vi "Setup Set Cluster Values from Pathed JSON String.vi"() -> (0 "error out":errorcluster, 2 "JSON string":string="{\n\t\"Width\":640,\n\t\"Height\":480,\n\t\"Sensor\":\"A700\",\n    \"TriggerMode\":0,\n    \"TriggerSource\":1,\n    \"TriggerActivation\":0,\n    \"TriggerSelector\":0,\n    \"AcquisitionMode\":2,\n    \"OutputImageType\":7,\n    \"AcquisitionFrameRate\":1.0,\n    \"AcquisitionFrameCount\":100,\n    \"Timeout\":20000,\n    \"FocusPos\":58000,\n    \"IncompleteBufferMode\":1,\n    \"IRFormat\":0,\n    \"NUCMode\":0,\n    \"NoiseReduction\":0\n}", 3 "specific class reference":refnum<vi>, 5 "path":string[](array[string]))   [LabVIEW 2023]
panel:
  out "Label.Text 2":string
  out "Label.Text":string
  in  "ClusterArray":T1(array[cluster]) {"Nested2"."IRFormat" items=["Option0", "Option1"]; "Nested1"."IRFormat" items=["Option0", "Option1"]}
  # "This VI is for Set Cluster Values from JSON String.lvtest"
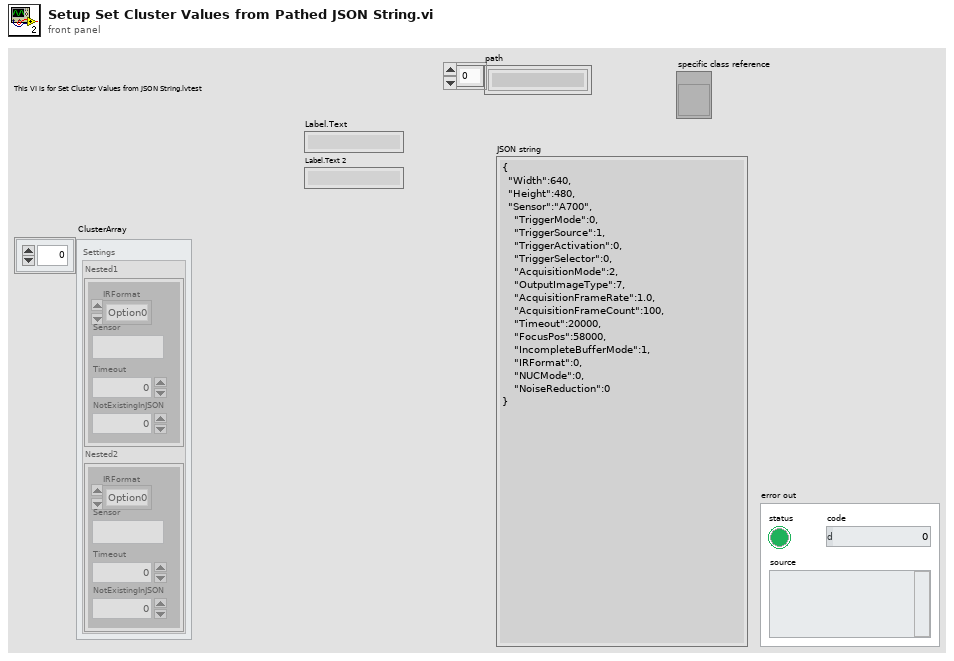
[diagram p1: front panel]
types:
  T1 = cluster{"Nested1":cluster{"IRFormat":u16, "Sensor":string, "Timeout":dbl, "NotExistingInJSON":dbl}, "Nested2":cluster{"IRFormat":u16, "Sensor":string, "Timeout":dbl, "NotExistingInJSON":dbl}}[]
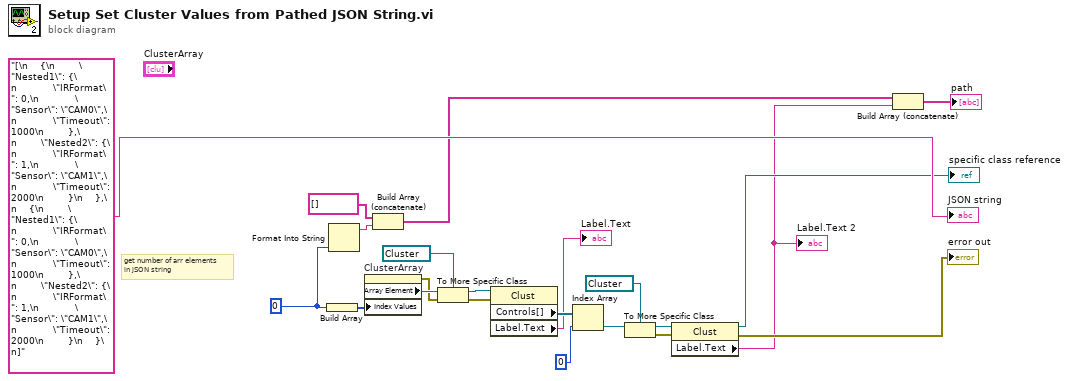
[diagram p0: block diagram]
diagram:
  w15 = 0 ("input 1")
  # "get number of arr elements\nin jSON string"
  n1 = Build Array(w15) -> (w17:i32[])
  n2 = Format Into String(w15) -> (resulting string=w21:string)  [unwired: 3 in, 1 out]
  n3 = property on="ClusterArray" class="Arr (strict)"("Index Values"=w17) -> (error out=w18:errorcluster, "Array Element"=w20:refnum<vi>)  [unwired: 2 in, 1 out]
  n4 = Build Array (concatenate)(string[] [], w21) -> (w10:string[])
  n5 = To More Specific Class(target class=refnum<vi> refnum ("specific class reference"), reference=w20, error in=w18) -> (specific class reference=w14:refnum<vi>, error out=w13:errorcluster)
  n6 = property class="Clust"(reference=w14, error in=w13) -> ("Controls[]"=w12:refnum<vi>[], "Label.Text"=→"Label.Text":string)  [unwired: 2 out]
  n7 = Index Array(array=w12, index=0) -> (element=w8:refnum<vi>)
  n8 = To More Specific Class(target class=refnum<vi> refnum ("specific class reference"), reference=w8) -> (specific class reference=w4:refnum<vi>, error out=w6:errorcluster)  [unwired: 1 in]
  n9 = property class="Clust"(reference=w4, error in=w6) -> (reference out=→"specific class reference":refnum<vi>, error out=→"error out":errorcluster, "Label.Text"=w2:string)
  "Label.Text 2" <- w2
  n10 = Build Array (concatenate)(w10, w2) -> (→"path":string[])
  "JSON string" <- "[\n    {\n        \"Nested1\": {\n            \"IRFormat\": 0,\n            \"Sensor\": \"CAM0\",\n            \"Timeout\": 1000\n        },\n        \"Nested2\": {\n            \"IRFormat\": 1,\n            \"Sensor\": \"CAM1\",\n            \"Timeout\": 2000\n        }\n    },\n    {\n        \"Nested1\": {\n            \"IRFormat\": 0,\n            \"Sensor\": \"CAM0\",\n            \"Timeout\": 1000\n        },\n        \"Nested2\": {\n            \"IRFormat\": 1,\n            \"Sensor\": \"CAM1\",\n            \"Timeout\": 2000\n        }\n    }\n]" ("JSON string")
